vi "toml_write_variant.vi"(7 "section":string[](array[string]), 8 "error in (no error)":errorcluster, 9 "value":variant, 10 "key":string[](array[string]), 11 "path in":path) -> (0 "error out":errorcluster, 2 "exists?":bool, 3 "path out":path)   [LabVIEW 2017]
uses:
  <vilib>/Utility/Data Type/NI_Data Type.lvlib
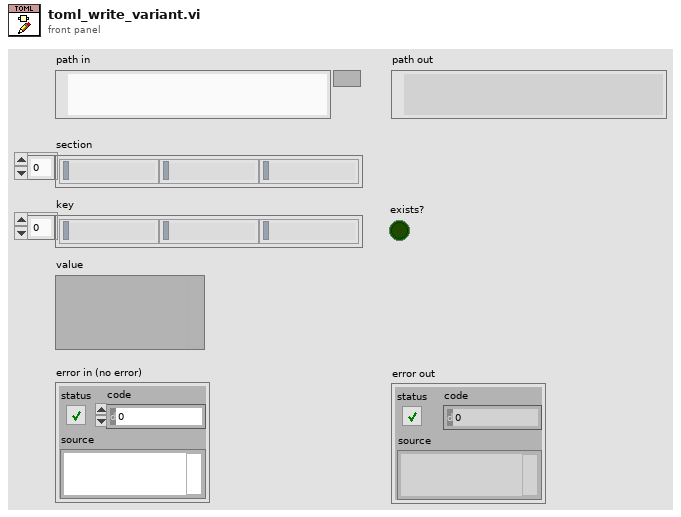
[diagram p1: front panel]
types:
  T1 = typedef "NI_Data Type.lvlib/Data Type.ctl" = enum8{"Invalid Type", "Void", "I8", "I16", "I32", "I64", "U8", "U16", "U32", "U64", "Single Float", "Double Float", "Extended Float", "Single Complex", "Double Complex", "Extended Complex", "Enum U8", "Enum U16", "Enum U32", "Enum U64", "Single Float With Unit", "Double Float With Unit", "Extended Float With Unit", "Single Complex with Unit", "Double Complex with Unit", "Extended Complex with Unit", "Boolean", "String", "Path", "Picture", "Tag", "Array", "Cluster", "Variant", "LV Variant", "Waveform", "Timestamp", "Digital Waveform", "Digital Data", "ExpressData", "Refnum", "External Data", "VI", "Poly VI", "LabVIEW Class Instance", "Fixed Point"}
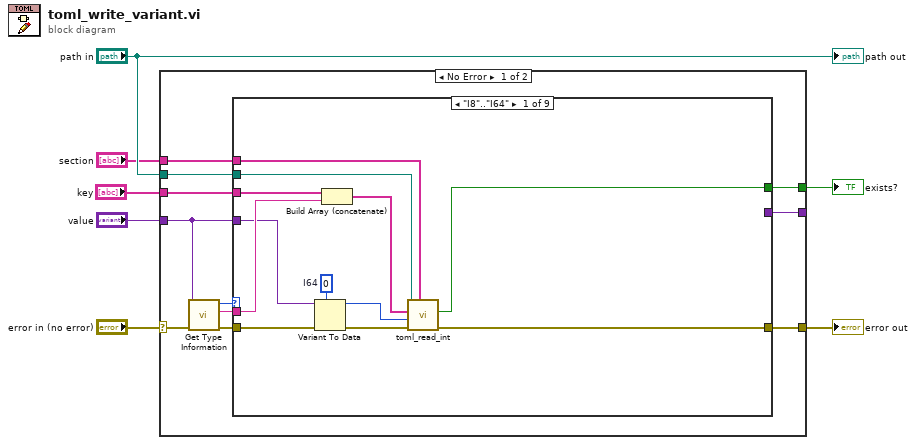
[diagram p0: block diagram]
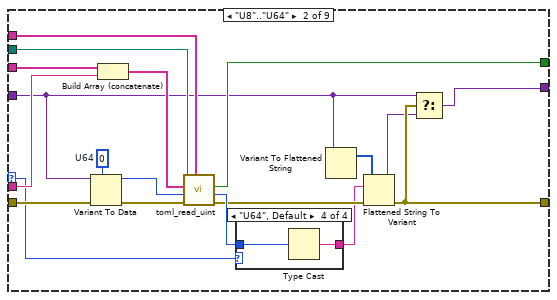
[diagram p2: hidden frame]
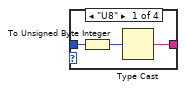
[diagram p3: hidden frame]
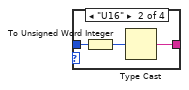
[diagram p4: hidden frame]
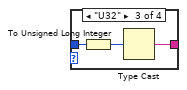
[diagram p5: hidden frame]
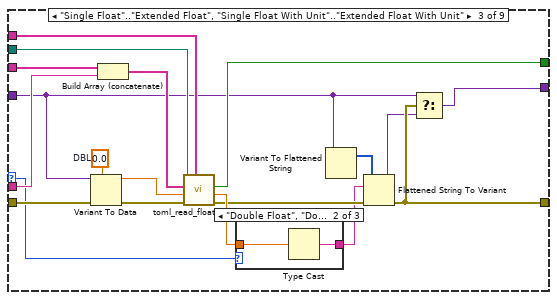
[diagram p6: hidden frame]
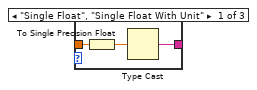
[diagram p7: hidden frame]
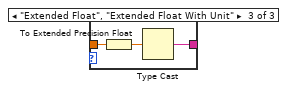
[diagram p8: hidden frame]
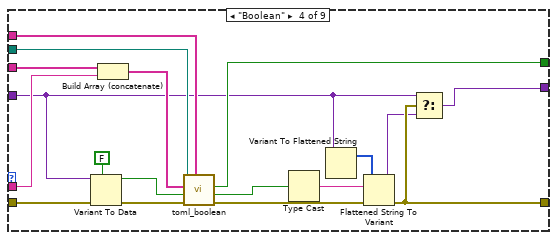
[diagram p9: hidden frame]
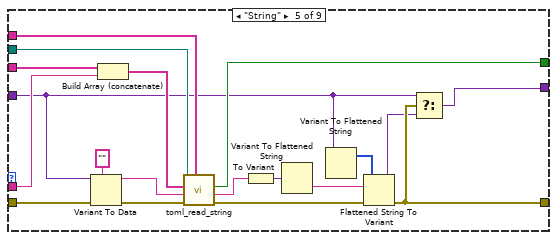
[diagram p10: hidden frame]
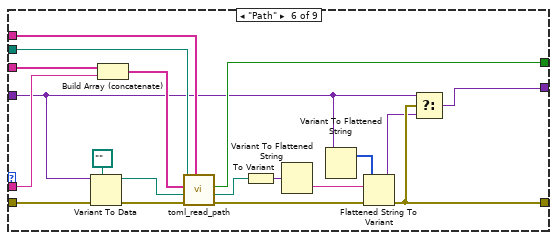
[diagram p11: hidden frame]
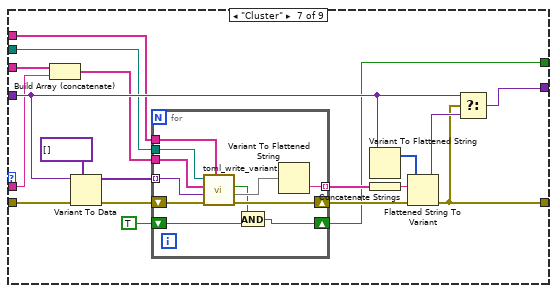
[diagram p12: hidden frame]
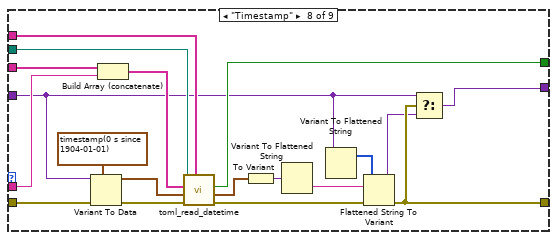
[diagram p13: hidden frame]
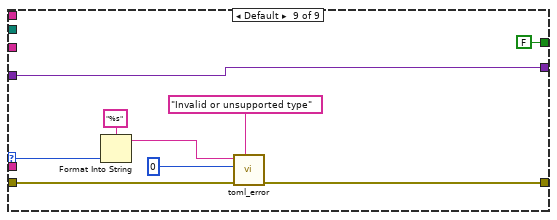
[diagram p14: hidden frame]
diagram:
  n1 = case shown="No Error" "error in (no error)" {
    selector: "error in (no error)" -> [w18 w204]
    tunnel: [w19 w204] -> w8
    tunnel: "value" -> [w16 w203]
    tunnel: [w14 w203] -> w5
    tunnel: "path in" -> [w13 _]
    tunnel: "section" -> [w11 _]
    tunnel: "key" -> [w10 _]
    tunnel: [w9 _] -> w1
    frame No Error {
      n2 = call <vilib>:"Get Type Information.vi"("error in (no error)"=w18, "Variant"=w16) -> ("error out"=w17:errorcluster, "Name"=w12:string, "Type"=w15:T1)  [unwired: 5 in, 2 out]
      n3 = case shown="\"I8\"..\"I64\"" w15 {
        selector: w15 -> [_ w37 w67 _ _ _ _ _ w198]
        tunnel: [w20 w35 w65 w92 w113 w132 w157 w181 w201] -> w19
        tunnel: w17 -> [w31 w50 w80 w106 w125 w144 w163 w193 w202]
        tunnel: w16 -> [w21 w34 w64 w91 w112 w131 w155 w180 w195]
        tunnel: [_ w32 w62 w89 w110 w129 w156 w178 w195] -> w14
        tunnel: w13 -> [w30 w49 w79 w105 w124 w143 w151 w192 _]
        tunnel: w12 -> [w27 w46 w76 w102 w121 w140 w153 w189 _]
        tunnel: w11 -> [w29 w48 w78 w104 w123 w142 w150 w191 _]
        tunnel: w10 -> [w28 w47 w77 w103 w122 w141 w154 w190 _]
        tunnel: [w22 w41 w71 w97 w116 w135 w145 w184 FALSE ("exists?")] -> w9
        frame "I8".."I64" {
          w24 = i64 0  # I64
          n4 = Variant To Data(error in=w31, type=w24, Variant=w21) -> (data=w23:i64, error out=w25:errorcluster)
          n5 = Build Array (concatenate)(w28, w27) -> (w26:string[])
          n6 = call "toml_read_int.vi"("section"=w29, "error in (no error)"=w25, "default"=w23, "key"=w26, "path in"=w30) -> ("error out"=w20:errorcluster, "exists?"=w22:bool)  [unwired: 3 in, 2 out]
        }
        frame "U8".."U64" {
          w43 = u64 0  # U64
          n7 = Variant To Data(error in=w50, type=w43, Variant=w34) -> (data=w42:u64, error out=w44:errorcluster)
          n8 = Build Array (concatenate)(w47, w46) -> (w45:string[])
          n9 = call "toml_read_uint.vi"("section"=w48, "error in (no error)"=w44, "default"=w42, "key"=w45, "path in"=w49) -> ("error out"=w39:errorcluster, "value"=w40:u64, "exists?"=w41:bool)  [unwired: 3 in, 1 out]
          n10 = case shown="\"U64\", Default" w37 {
            tunnel: [w51 w54 w57 w61] -> w36
            tunnel: w40 -> [w53 w56 w59 w60]
            frame "U8" {
              n11 = To Unsigned Byte Integer(number=w53) -> (unsigned 8bit integer=w52:u8)
              n12 = Type Cast(x=w52) -> (*(type *) &x=w51:string)  [unwired: 1 in]
            }
            frame "U16" {
              n13 = To Unsigned Word Integer(number=w56) -> (unsigned 16bit integer=w55:u16)
              n14 = Type Cast(x=w55) -> (*(type *) &x=w54:string)  [unwired: 1 in]
            }
            frame "U32" {
              n15 = To Unsigned Long Integer(number=w59) -> (unsigned 32bit integer=w58:u32)
              n16 = Type Cast(x=w58) -> (*(type *) &x=w57:string)  [unwired: 1 in]
            }
            frame "U64", Default {
              n17 = Type Cast(x=w60) -> (*(type *) &x=w61:string)  [unwired: 1 in]
            }
          }
          n18 = Variant To Flattened String(Variant=w34) -> (1:w38:i16[])  [unwired: 1 out]
          n19 = Flattened String To Variant(4:w39, 6:w36, 7:w38) -> (0:w35:errorcluster, 3:w33:variant)
          n20 = Select(t=w34, s=w35, f=w33) -> (s? t:f=w32:variant)
        }
        frame "Single Float".."Extended Float", "Single Float With Unit".."Extended Float With Unit" {
          w73 = 0.0  # DBL
          n21 = Variant To Data(error in=w80, type=w73, Variant=w64) -> (data=w72:dbl, error out=w74:errorcluster)
          n22 = Build Array (concatenate)(w77, w76) -> (w75:string[])
          n23 = call "toml_read_float.vi"("section"=w78, "error in (no error)"=w74, "default"=w72, "key"=w75, "path in"=w79) -> ("error out"=w69:errorcluster, "value"=w70:dbl, "exists?"=w71:bool)  [unwired: 3 in, 1 out]
          n24 = case shown="\"Double Float\", \"Double Float With Unit\", Default" w67 {
            tunnel: [w81 w85 w88] -> w66
            tunnel: w70 -> [w83 w84 w87]
            frame "Single Float", "Single Float With Unit" {
              n25 = To Single Precision Float(number=w83) -> (single precision float=w82:sgl)
              n26 = Type Cast(x=w82) -> (*(type *) &x=w81:string)  [unwired: 1 in]
            }
            frame "Double Float", "Double Float With Unit", Default {
              n27 = Type Cast(x=w84) -> (*(type *) &x=w85:string)  [unwired: 1 in]
            }
            frame "Extended Float", "Extended Float With Unit" {
              n28 = To Extended Precision Float(1:w87) -> (0:w86:ext)
              n29 = Type Cast(x=w86) -> (*(type *) &x=w88:string)  [unwired: 1 in]
            }
          }
          n30 = Variant To Flattened String(Variant=w64) -> (1:w68:i16[])  [unwired: 1 out]
          n31 = Flattened String To Variant(4:w69, 6:w66, 7:w68) -> (0:w65:errorcluster, 3:w63:variant)
          n32 = Select(t=w64, s=w65, f=w63) -> (s? t:f=w62:variant)
        }
        frame "Boolean" {
          n33 = Variant To Data(error in=w106, type=FALSE, Variant=w91) -> (data=w98:bool, error out=w100:errorcluster)
          n34 = Build Array (concatenate)(w103, w102) -> (w101:string[])
          n35 = call "toml_boolean.vi"("section"=w104, "error in (no error)"=w100, "default"=w98, "key"=w101, "path in"=w105) -> ("error out"=w95:errorcluster, "value"=w96:bool, "exists?"=w97:bool)  [unwired: 3 in, 1 out]
          n36 = Type Cast(x=w96) -> (*(type *) &x=w93:string)  [unwired: 1 in]
          n37 = Variant To Flattened String(Variant=w91) -> (1:w94:i16[])  [unwired: 1 out]
          n38 = Flattened String To Variant(4:w95, 6:w93, 7:w94) -> (0:w92:errorcluster, 3:w90:variant)
          n39 = Select(t=w91, s=w92, f=w90) -> (s? t:f=w89:variant)
        }
        frame "String" {
          n40 = Variant To Data(error in=w125, type="", Variant=w112) -> (data=w117:string, error out=w119:errorcluster)
          n41 = Build Array (concatenate)(w122, w121) -> (w120:string[])
          n42 = call "toml_read_string.vi"("section"=w123, "error in (no error)"=w119, "default"=w117, "key"=w120, "path in"=w124) -> ("error out"=w115:errorcluster, "value"=w109:string, "exists?"=w116:bool)  [unwired: 3 in, 1 out]
          n43 = To Variant(anything=w109) -> (Variant=w107:variant)
          n44 = Variant To Flattened String(Variant=w107) -> (data string=w108:string)  [unwired: 1 out]
          n45 = Variant To Flattened String(Variant=w112) -> (1:w114:i16[])  [unwired: 1 out]
          n46 = Flattened String To Variant(4:w115, 6:w108, 7:w114) -> (0:w113:errorcluster, 3:w111:variant)
          n47 = Select(t=w112, s=w113, f=w111) -> (s? t:f=w110:variant)
        }
        frame "Path" {
          n48 = Variant To Data(error in=w144, type=path "", Variant=w131) -> (data=w136:path, error out=w138:errorcluster)
          n49 = Build Array (concatenate)(w141, w140) -> (w139:string[])
          n50 = call "toml_read_path.vi"("section"=w142, "error in (no error)"=w138, "default"=w136, "key"=w139, "path in"=w143) -> ("error out"=w134:errorcluster, "value"=w128:path, "exists?"=w135:bool)  [unwired: 3 in, 1 out]
          n51 = To Variant(anything=w128) -> (Variant=w126:variant)
          n52 = Variant To Flattened String(Variant=w126) -> (data string=w127:string)  [unwired: 1 out]
          n53 = Variant To Flattened String(Variant=w131) -> (1:w133:i16[])  [unwired: 1 out]
          n54 = Flattened String To Variant(4:w134, 6:w127, 7:w133) -> (0:w132:errorcluster, 3:w130:variant)
          n55 = Select(t=w131, s=w132, f=w130) -> (s? t:f=w129:variant)
        }
        frame "Cluster" {
          n56 = Build Array (concatenate)(w154, w153) -> (w152:string[])
          n57 = Variant To Data(error in=w163, type=variant[] [], Variant=w155) -> (data=w149:variant[], error out=w161:errorcluster)
          n58 = for {
            shift-right: [w173] -> w158
            shift-left: w161 -> [w174]
            tunnel: w152 -> [w172]
            tunnel: w151 -> [w171]
            tunnel: w150 -> [w170]
            tunnel: w149 -> [w169] mode=indexing
            tunnel: [w167] -> w148 mode=indexing
            shift-right: [w164] -> w145
            shift-left: TRUE -> [w165]
            n59 = call "toml_write_variant.vi"("section"=w170, "error in (no error)"=w174, "value"=w169, "key"=w172, "path in"=w171) -> ("error out"=w173:errorcluster, 1:w168, "exists?"=w166:bool)  [unwired: 3 in, 1 out]
            n60 = And(x=w166, y=w165) -> (x .and. y?=w164:bool)
            n61 = Variant To Flattened String(Variant=w168) -> (data string=w167:string)  [unwired: 1 out]
          }
          n62 = Variant To Flattened String(Variant=w155) -> (1:w160:i16[])  [unwired: 1 out]
          n63 = Concatenate Strings(w148) -> (w147:string)
          n64 = Flattened String To Variant(4:w158, 6:w147, 7:w160) -> (0:w157:errorcluster, 3:w159:variant)
          n65 = Select(t=w155, s=w157, f=w159) -> (s? t:f=w156:variant)
        }
        frame "Timestamp" {
          n66 = Variant To Data(error in=w193, type=timestamp(0 s since 1904-01-01), Variant=w180) -> (data=w185:timestamp, error out=w187:errorcluster)
          n67 = Build Array (concatenate)(w190, w189) -> (w188:string[])
          n68 = call "toml_read_datetime.vi"("section"=w191, "error in (no error)"=w187, "default"=w185, "key"=w188, "path in"=w192) -> ("error out"=w183:errorcluster, "value"=w177:timestamp, "exists?"=w184:bool)  [unwired: 3 in, 1 out]
          n69 = To Variant(anything=w177) -> (Variant=w175:variant)
          n70 = Variant To Flattened String(Variant=w175) -> (data string=w176:string)  [unwired: 1 out]
          n71 = Variant To Flattened String(Variant=w180) -> (1:w182:i16[])  [unwired: 1 out]
          n72 = Flattened String To Variant(4:w183, 6:w176, 7:w182) -> (0:w181:errorcluster, 3:w179:variant)
          n73 = Select(t=w180, s=w181, f=w179) -> (s? t:f=w178:variant)
        }
        frame Default {
          n74 = Format Into String(format string="%s", w198) -> (resulting string=w196:string)  [unwired: 2 in, 1 out]
          n75 = call "toml_error.vi"("message"="Invalid or unsupported type", "error in (no error)"=w202, "offset (0)"=0, "toml"=w196) -> ("error out"=w201:errorcluster)  [unwired: 7 in]
        }
      }
    }
    frame Error {
    }
  }
  "error out" <- w8
  "exists?" <- w1
  "path out" <- "path in"
